vi "iRobot SensorGroup6 to Stream.vi"(11 "iRobot Sensor Group 6":T1={"Bumps + Wheel Drops"={"Wheeldrop Caster"=FALSE, "Wheeldrop Left"=FALSE, "Wheeldrop Right"=FALSE, "Bump Left"=FALSE, "Bump Right"=FALSE}, "Wall"=FALSE, "Cliff Left"=FALSE, "Cliff Front Left"=FALSE, "Cliff Front Right"=FALSE, "Cliff Right"=FALSE, "Wall Signal"=0, "Cliff Left Signal"=0, "Cliff Front Left Signal"=0, "Cliff Front Right Signal"=0, "Cliff Right Signal"=0, "Buttons"={"Advance"=FALSE, "Play"=FALSE}, "Virtual Wall"=FALSE, "# Stream Packets"=0, "Requested Velocity (mm/s)"=0, "Requested Radius (mm)"=0, "Requested Right Wheel Velocity (mm/s)"=0, "Requested Left Wheel Velocity (mm/s)"=0, "Distance (mm)"=0, "Angle (deg)"=0, "Song Playing"=FALSE, "Song Number"=0, "Charging State"=enum."Not Charging", "Voltage (mV)"=0, "Current (mA)"=0, "Battery Temperature (deg C)"=0, "Battery Charge (mAh)"=0, "Battery Capacity (mAh)"=0, "Charging Sources"={"Internal Charger"=FALSE, "Home Base"=FALSE}, "OI Mode"=enum."Off", "Digital Inputs"={"Digital Input 0"=FALSE, "Digital Input 1"=FALSE, "Digital Input 2"=FALSE, "Digital Input 3"=FALSE, "Device Detect"=FALSE}, "Drivers & Wheel Overcurrent"={"Low-Side Driver 0"=FALSE, "Low-Side Driver 1"=FALSE, "Low-Side Driver 2"=FALSE, "Left Wheel"=FALSE, "Right Wheel"=FALSE}, "Analog Signal"=0, "Infrared"=255} {"Infrared" format="%02x"}) -> (2 "packet":u8[](array[numeric]), 3 "stream":u8[](array[numeric]))   [LabVIEW 2014]
uses:
  Sensor Group 6.ctl
  Bumps + Wheel Drops.ctl
  Buttons.ctl
  Charging State.ctl
  Charging Sources Available.ctl
  OI Mode.ctl
  Cargo Bay Digital Inputs.ctl
  Low-Side Driver + Wheel Overcurrent.ctl
panel:
  # "Electrical: charging, battery, OI mode"
  # "Sensors: bump, cliff, button, wheel drop, wall, virtual wall"
  # "Motion: distance, angle, requested velocity"
  # "Cargo Bay: I/O, overcurrent, infrared"
  # "Song"
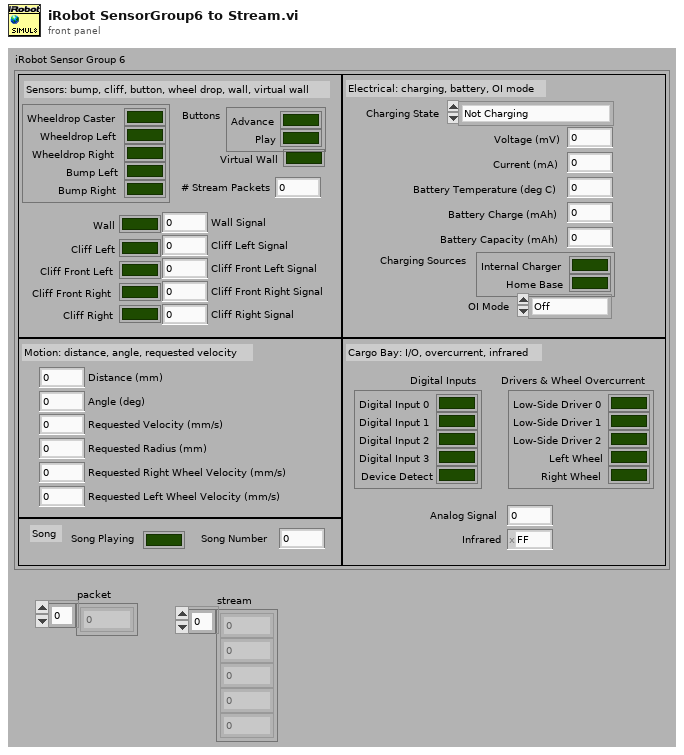
[diagram p1: front panel]
types:
  T1 = typedef "Sensor Group 6.ctl" = cluster{"Bumps + Wheel Drops":T2, "Wall":bool, "Cliff Left":bool, "Cliff Front Left":bool, "Cliff Front Right":bool, "Cliff Right":bool, "Wall Signal":u16, "Cliff Left Signal":u16, "Cliff Front Left Signal":u16, "Cliff Front Right Signal":u16, "Cliff Right Signal":u16, "Buttons":T3, "Virtual Wall":bool, "# Stream Packets":u8, "Requested Velocity (mm/s)":i16, "Requested Radius (mm)":i16, "Requested Right Wheel Velocity (mm/s)":i16, "Requested Left Wheel Velocity (mm/s)":i16, "Distance (mm)":i32, "Angle (deg)":i32, "Song Playing":bool, "Song Number":u8, "Charging State":T4, "Voltage (mV)":u16, "Current (mA)":i16, "Battery Temperature (deg C)":i8, "Battery Charge (mAh)":u16, "Battery Capacity (mAh)":u16, "Charging Sources":T5, "OI Mode":T6, "Digital Inputs":T7, "Drivers & Wheel Overcurrent":T8, "Analog Signal":u16, "Infrared":u8}
  T2 = typedef "Bumps + Wheel Drops.ctl" = cluster{"Wheeldrop Caster":bool, "Wheeldrop Left":bool, "Wheeldrop Right":bool, "Bump Left":bool, "Bump Right":bool}
  T3 = typedef "Buttons.ctl" = cluster{"Advance":bool, "Play":bool}
  T4 = typedef "Charging State.ctl" = enum16{"Not Charging", "Reconditioning Charging", "Full Charging", "Trickle Charging", "Waiting", "Charging Fault Condition"}
  T5 = typedef "Charging Sources Available.ctl" = cluster{"Internal Charger":bool, "Home Base":bool}
  T6 = typedef "OI Mode.ctl" = enum16{"Off", "Passive", "Safe", "Full"}
  T7 = typedef "Cargo Bay Digital Inputs.ctl" = cluster{"Digital Input 0":bool, "Digital Input 1":bool, "Digital Input 2":bool, "Digital Input 3":bool, "Device Detect":bool}
  T8 = typedef "Low-Side Driver + Wheel Overcurrent.ctl" = cluster{"Low-Side Driver 0":bool, "Low-Side Driver 1":bool, "Low-Side Driver 2":bool, "Left Wheel":bool, "Right Wheel":bool}
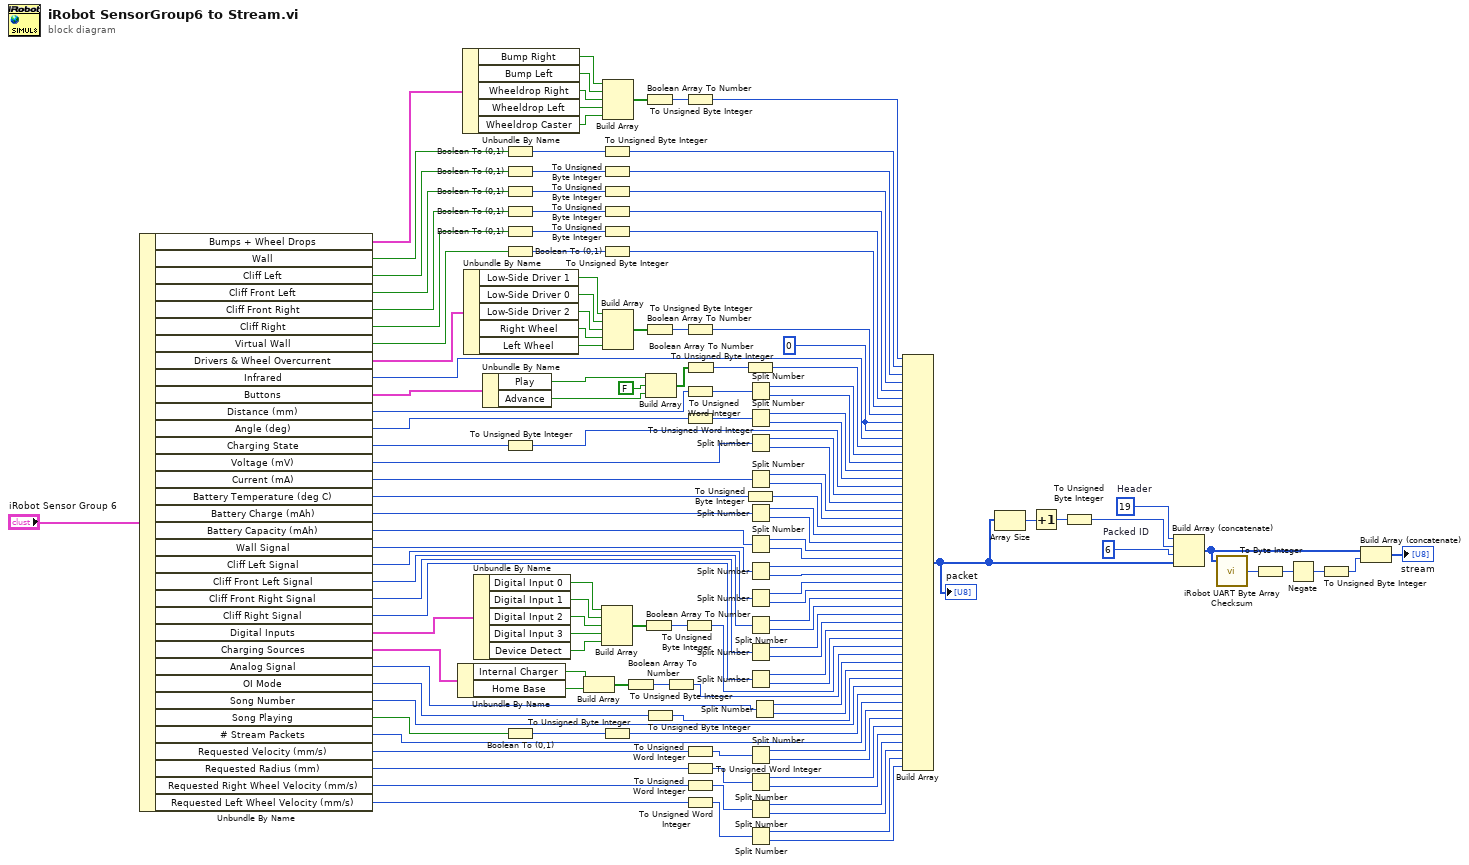
[diagram p0: block diagram]
diagram:
  w12 = u8 6  # Packed ID
  w17 = u8 19  # Header
  w99 = u8 0 ("element")
  n1 = Unbundle By Name("iRobot Sensor Group 6") -> ("Bumps + Wheel Drops"=w137:T2, "Wall"=w122:bool, "Cliff Left"=w121:bool, "Cliff Front Left"=w123:bool, "Cliff Front Right"=w124:bool, "Cliff Right"=w125:bool, "Virtual Wall"=w126:bool, "Drivers & Wheel Overcurrent"=w136:T8, "Infrared"=w98:u8, "Buttons"=w135:T3, "Distance (mm)"=w90:i32, "Angle (deg)"=w86:i32, "Charging State"=w83:T4, "Voltage (mV)"=w81:u16, "Current (mA)"=w78:i16, "Battery Temperature (deg C)"=w75:i8, "Battery Charge (mAh)"=w73:u16, "Battery Capacity (mAh)"=w70:u16, "Wall Signal"=w67:u16, "Cliff Left Signal"=w66:u16, "Cliff Front Left Signal"=w65:u16, "Cliff Front Right Signal"=w64:u16, "Cliff Right Signal"=w63:u16, "Digital Inputs"=w134:T7, "Charging Sources"=w2:T5, "Analog Signal"=w1:u16, "OI Mode"=w40:T6, "Song Number"=w38:u8, "Song Playing"=w37:bool, "# Stream Packets"=w34:u8, "Requested Velocity (mm/s)"=w32:i16, "Requested Radius (mm)"=w29:i16, "Requested Right Wheel Velocity (mm/s)"=w25:i16, "Requested Left Wheel Velocity (mm/s)"=w21:i16)
  n2 = Unbundle By Name(w2) -> ("Internal Charger"=w44:bool, "Home Base"=w43:bool)
  n3 = Unbundle By Name(w137) -> ("Bump Right"=w133:bool, "Bump Left"=w132:bool, "Wheeldrop Right"=w131:bool, "Wheeldrop Left"=w130:bool, "Wheeldrop Caster"=w108:bool)
  n4 = Unbundle By Name(w136) -> ("Low-Side Driver 1"=w107:bool, "Low-Side Driver 0"=w106:bool, "Low-Side Driver 2"=w105:bool, "Right Wheel"=w104:bool, "Left Wheel"=w103:bool)
  n5 = Unbundle By Name(w134) -> ("Digital Input 0"=w52:bool, "Digital Input 1"=w51:bool, "Digital Input 2"=w50:bool, "Digital Input 3"=w49:bool, "Device Detect"=w48:bool)
  n6 = Unbundle By Name(w135) -> ("Play"=w97:bool, "Advance"=w95:bool)
  n7 = Boolean To (0,1)(Boolean=w122) -> (0, 1=w120:i16)
  n8 = Boolean To (0,1)(Boolean=w121) -> (0, 1=w115:i16)
  n9 = Boolean To (0,1)(Boolean=w123) -> (0, 1=w116:i16)
  n10 = Boolean To (0,1)(Boolean=w124) -> (0, 1=w117:i16)
  n11 = Boolean To (0,1)(Boolean=w125) -> (0, 1=w118:i16)
  n12 = Boolean To (0,1)(Boolean=w126) -> (0, 1=w119:i16)
  n13 = To Unsigned Byte Integer(number=w83) -> (unsigned 8bit integer=w82:u8)
  n14 = Boolean To (0,1)(Boolean=w37) -> (0, 1=w36:i16)
  n15 = Build Array(w44, w43) -> (w41:bool[])
  n16 = To Unsigned Byte Integer(number=w120) -> (unsigned 8bit integer=w114:u8)
  n17 = To Unsigned Byte Integer(number=w115) -> (unsigned 8bit integer=w113:u8)
  n18 = To Unsigned Byte Integer(number=w116) -> (unsigned 8bit integer=w112:u8)
  n19 = To Unsigned Byte Integer(number=w117) -> (unsigned 8bit integer=w111:u8)
  n20 = To Unsigned Byte Integer(number=w118) -> (unsigned 8bit integer=w110:u8)
  n21 = To Unsigned Byte Integer(number=w119) -> (unsigned 8bit integer=w109:u8)
  n22 = Build Array(w52, w51, w50, w49, w48) -> (w46:bool[])
  n23 = To Unsigned Byte Integer(number=w36) -> (unsigned 8bit integer=w35:u8)
  n24 = Build Array(w133, w132, w131, w130, w108) -> (w129:bool[])
  n25 = Build Array(w107, w106, w105, w104, w103) -> (w101:bool[])
  n26 = Boolean Array To Number(Boolean array=w41) -> (number=w42:u32)
  n27 = Boolean Array To Number(Boolean array=w46) -> (number=w47:u32)
  n28 = Boolean Array To Number(Boolean array=w129) -> (number=w128:u32)
  n29 = Boolean Array To Number(Boolean array=w101) -> (number=w102:u32)
  n30 = To Unsigned Byte Integer(number=w40) -> (unsigned 8bit integer=w39:u8)
  n31 = Build Array(w97, FALSE ("element"), w95) -> (w93:bool[])
  n32 = To Unsigned Byte Integer(number=w42) -> (unsigned 8bit integer=w3:u8)
  n33 = To Unsigned Byte Integer(number=w47) -> (unsigned 8bit integer=w45:u8)
  n34 = To Unsigned Byte Integer(number=w128) -> (unsigned 8bit integer=w127:u8)
  n35 = To Unsigned Byte Integer(number=w102) -> (unsigned 8bit integer=w100:u8)
  n36 = To Unsigned Word Integer(number=w90) -> (unsigned 16bit integer=w91:u16)
  n37 = To Unsigned Word Integer(number=w86) -> (unsigned 16bit integer=w87:u16)
  n38 = To Unsigned Word Integer(number=w32) -> (unsigned 16bit integer=w33:u16)
  n39 = To Unsigned Word Integer(number=w29) -> (unsigned 16bit integer=w28:u16)
  n40 = To Unsigned Word Integer(number=w25) -> (unsigned 16bit integer=w24:u16)
  n41 = To Unsigned Word Integer(number=w21) -> (unsigned 16bit integer=w20:u16)
  n42 = Boolean Array To Number(Boolean array=w93) -> (number=w94:u32)
  n43 = To Unsigned Byte Integer(number=w94) -> (unsigned 8bit integer=w92:u8)
  n44 = To Unsigned Byte Integer(number=w75) -> (unsigned 8bit integer=w74:u8)
  n45 = Split Number(x=w91) -> (hi(x)=w89:u8, lo(x)=w88:u8)
  n46 = Split Number(x=w87) -> (hi(x)=w85:u8, lo(x)=w84:u8)
  n47 = Split Number(x=w81) -> (hi(x)=w80:u8, lo(x)=w79:u8)
  n48 = Split Number(x=w78) -> (hi(x)=w77:u8, lo(x)=w76:u8)
  n49 = Split Number(x=w73) -> (hi(x)=w72:u8, lo(x)=w71:u8)
  n50 = Split Number(x=w70) -> (hi(x)=w69:u8, lo(x)=w68:u8)
  n51 = Split Number(x=w67) -> (hi(x)=w62:u8, lo(x)=w61:u8)
  n52 = Split Number(x=w66) -> (hi(x)=w60:u8, lo(x)=w59:u8)
  n53 = Split Number(x=w65) -> (hi(x)=w58:u8, lo(x)=w57:u8)
  n54 = Split Number(x=w64) -> (hi(x)=w56:u8, lo(x)=w55:u8)
  n55 = Split Number(x=w63) -> (hi(x)=w54:u8, lo(x)=w53:u8)
  n56 = Split Number(x=w33) -> (hi(x)=w31:u8, lo(x)=w30:u8)
  n57 = Split Number(x=w28) -> (hi(x)=w27:u8, lo(x)=w26:u8)
  n58 = Split Number(x=w24) -> (hi(x)=w23:u8, lo(x)=w22:u8)
  n59 = Split Number(x=w20) -> (hi(x)=w19:u8, lo(x)=w18:u8)
  n60 = Split Number(x=w1) -> (hi(x)=w4:u8, lo(x)=w5:u8)
  n61 = Build Array(w127, w114, w113, w112, w111, w110, w109, w100, w99, w99, w98, w92, w89, w88, w85, w84, w82, w80, w79, w77, w76, w74, w72, w71, w69, w68, w62, w61, w60, w59, w58, w57, w56, w55, w54, w53, w45, w3, w4, w5, w39, w38, w35, w34, w31, w30, w27, w26, w23, w22, w19, w18) -> (w10:u8[])
  "packet" <- w10
  n62 = Array Size(array=w10) -> (size(s)=w16:i32)
  n63 = Increment(x=w16) -> (x+1=w15:i32)
  n64 = To Unsigned Byte Integer(number=w15) -> (unsigned 8bit integer=w14:u8)
  n65 = Build Array (concatenate)(w17, w14, w12, w10) -> (w13:u8[])
  n66 = call "iRobot UART Byte Array Checksum.vi"("Byte Array"=w13) -> ("Checksum"=w9:u8)  [unwired: 2 in]
  n67 = To Byte Integer(number=w9) -> (8bit integer=w8:i8)
  n68 = Negate(x=w8) -> (-x=w6:i8)
  n69 = To Unsigned Byte Integer(number=w6) -> (unsigned 8bit integer=w7:u8)
  n70 = Build Array (concatenate)(w13, w7) -> (→"stream":u8[])
